vi "Update Log Directory.vi"(0 "reference in":refnum<class "Logger.lvclass">, 2 "Log Directory":path, 5 "Error In":errorcluster) -> (14 "reference out":refnum<class "Logger.lvclass">, 19 "Error Out":errorcluster)   [LabVIEW 2023, in "Logger.lvclass"]
uses:
  Logger.lvclass
  Logger.lvclass/Logger.ctl
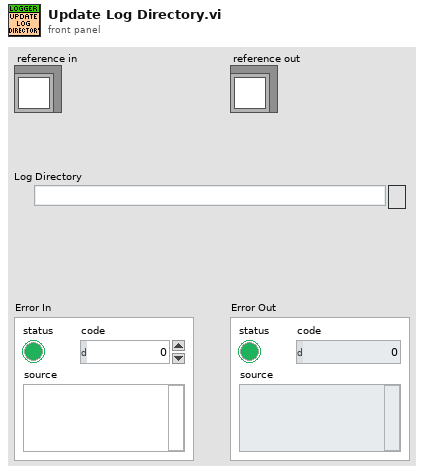
[diagram p1: front panel]
types:
  T1 = typedef "Logger.lvclass/ObjectAttributes.ctl" = cluster{"Output Directory":path, "Log File Type":enum16{"TDMS", "CSV"}, "Logger Queue":refnum<queue>, "HPS17K Refs":refnum<class "HPS-17000.lvclass">[]}
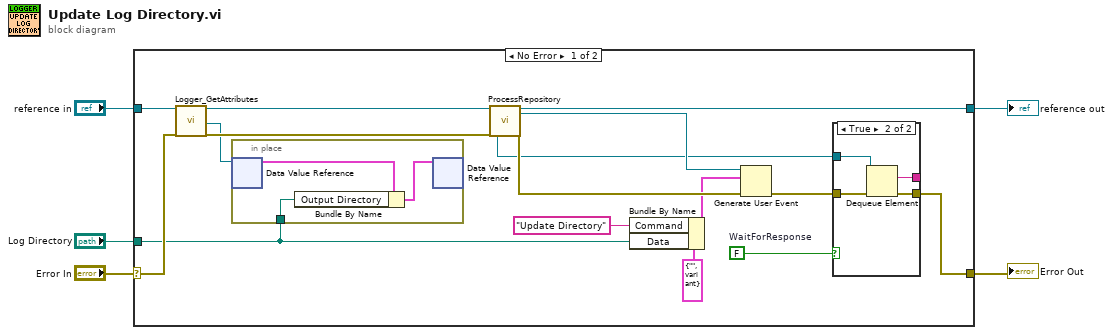
[diagram p0: block diagram]
diagram:
  n1 = case shown="No Error" "Error In" {
    selector: "Error In" -> [w8 w31]
    tunnel: [w16 w31] -> w4
    tunnel: [w21 w30] -> w2
    tunnel: "reference in" -> [w11 w30]
    tunnel: "Log Directory" -> [w6 _]
    frame No Error {
      w19 = FALSE  # WaitForResponse
      n2 = call "Logger_GetAttributes.vi"("reference in"=w11, "Error In"=w8) -> ("reference out"=w10:refnum<class "Logger.lvclass">, "DataRef"=w7:refnum<data-value>, "Error Out"=w9:errorcluster)  [unwired: 14 in, 1 out]
      n3 = in-place {
        in-place-border: w6 -> [w22]
        n4 = in-place-dvr #1(w7) -> (w24:T1)  [unwired: 1 out]
        n5 = Bundle By Name(cluster=w24, "Output Directory"=w22) -> (w23:T1)
        n6 = in-place-dvr #1(w23) -> ()  [unwired: 2 out]
      }
      n7 = call "ProcessRepository.vi"("reference in"=w10, "Error In"=w9) -> ("QueueFromProcess"=w13:refnum<queue>, "reference out"=w21:refnum<class "Logger.lvclass">, "EventsToProcess"=w20:refnum<user-event>, "Error Out"=w17:errorcluster)  [unwired: 10 in, 4 out]
      n8 = Bundle By Name(cluster=cluster{"Command":string, "Data":variant} {"Command"="", "Data"=variant} ("MessageToProcess"), "Command"="Update Directory", "Data"=w6) -> (w14:cluster{"Command":string, "Data":variant})
      n9 = Generate User Event(user event=w20, event data cluster=w14, error in=w17) -> (error out=w18:errorcluster)  [unwired: 1 in, 1 out]
      n10 = case shown="True" w19 {
        tunnel: w18 -> [w25 w29]
        tunnel: [_ w28] -> _
        tunnel: [w25 w27] -> w16
        tunnel: w13 -> [_ w26]
        frame False {
        }
        frame True {
          n11 = Dequeue Element(queue=w26, error in (no error)=w29) -> (element=w28:string, error out=w27:errorcluster)  [unwired: 1 in, 2 out]
        }
      }
    }
    frame Error {
    }
  }
  "Error Out" <- w4
  "reference out" <- w2
